vi "get_pos.vi"(8 "error in (no error)":errorcluster caption="错误输入（无错误）", 11 "StepMotor 输入":refnum<class "StepMotor.lvclass">) -> (0 "error out":errorcluster caption="错误输出", 2 "pos":i32, 3 "StepMotor 输出":refnum<class "StepMotor.lvclass">)   [LabVIEW 2016, in "MotionControl_UFO_3DOF.lvlib" / "StepMotor.lvclass"]
uses:
  <userlib>/MotionControl_UFO_3DOF/StepMotor/StepMotor.lvclass
  <userlib>/MotionControl_UFO_3DOF/StepMotor/StepMotor.lvclass/StepMotor.ctl
  <userlib>/UISimCanFunc_wrapper/UISimCanFunc_wrapper.lvlib
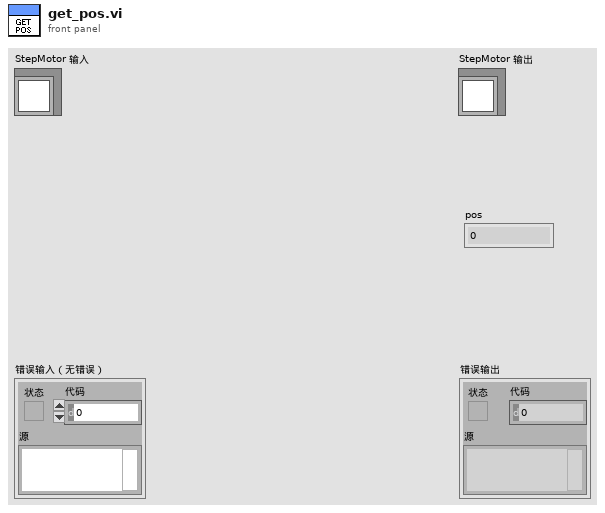
[diagram p1: front panel]
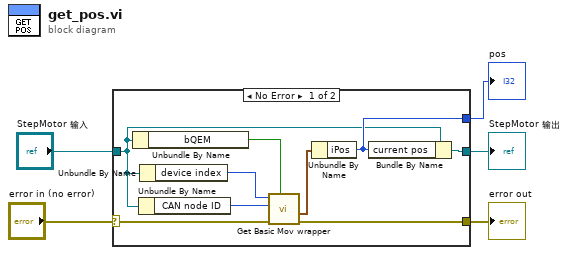
[diagram p0: block diagram]
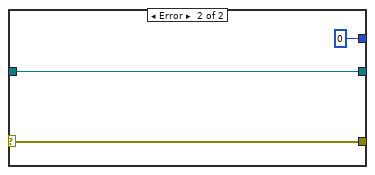
[diagram p2: hidden frame]
diagram:
  n1 = case shown="No Error" "error in (no error)" {
    selector: "error in (no error)" -> [w11 w17]
    tunnel: [w10 w17] -> w4
    tunnel: [w6 w16] -> w2
    tunnel: "StepMotor 输入" -> [w7 w16]
    tunnel: [w8 0] -> w1
    frame No Error {
      n2 = Unbundle By Name(w7) -> ("bQEM"=w14:bool)
      n3 = Unbundle By Name(w7) -> ("CAN node ID"=w12:u32)
      n4 = Unbundle By Name(w7) -> ("device index"=w13:u32)
      n5 = call <userlib>:"Get Basic Mov wrapper.vi"("bLoop"=w14, "error in (no error)"=w11, "dwCanNodeId"=w12, "dwDevIndex"=w13) -> ("error out"=w10:errorcluster, "pBasicMovObj out"=w9:cluster{"iSpd":i32, "iPos":i32, "iTimeOut":i32})  [unwired: 5 in, 1 out]
      n6 = Unbundle By Name(w9) -> ("iPos"=w8:i32)
      n7 = Bundle By Name(cluster=w7, "current pos"=w8) -> (w6:refnum<class "StepMotor.lvclass">)
    }
    frame Error {
    }
  }
  "error out" <- w4
  "StepMotor 输出" <- w2
  "pos" <- w1
